vi "Demo2 (FPGA).vi"() -> ()   [LabVIEW 2023]
uses:
  Instance           1 20Saved   Demo2 (FPGA) .vi
  <vilib>/eio/EIONode/EIONode.xnode
  Instance           2 20Saved   Demo2 (FPGA) .vi
  <vilib>/rvi/DataTransferAndStorage/Container/XNode/niFpgaContainer.xnode
  <vilib>/rvi/eio/common/nirviEmuTemplateMethod_errors.vi
  <vilib>/rvi/FIFO/Fifo_Resource/nirvififoEmulationRead.vi
  <vilib>/rvi/FIFO/Fifo_Resource/nirvififoEmulationWrite.vi
panel:
  in  "Bypass interpolation filter?":bool
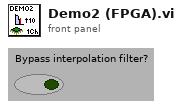
[diagram p1: front panel]
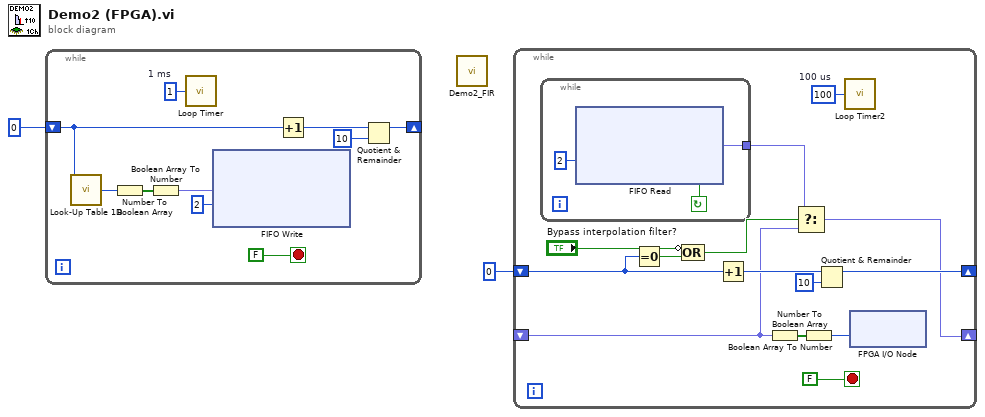
[diagram p0: block diagram]
diagram:
  n1 = while {
    shift-right: [w9] -> _
    shift-left: u8 0 -> [w8]
    stop <- FALSE stop-if-true
    w12 = u8 1  # 1 ms
    n2 = call "Look-Up Table 1D"("address"=w8) -> ("data out"=w7:i16)  [unwired: 8 in]
    n3 = Number To Boolean Array(number=w7) -> (Boolean array=w4:bool[])
    n4 = Boolean Array To Number(Boolean array=w4) -> (number=w3:fxp<+/-,16,1>)
    n5 = call "Loop Timer"("Count(mSec)"=w12) -> ()  [unwired: 1 out]
    n6 = xnode ("FIFO Write")("Element"=w3, "Timeout"=2) -> ()  [unwired: 1 in, 2 out]
    n7 = Increment(x=w8) -> (x+1=w11:u8)
    n8 = Quotient & Remainder(x=w11, y=u8 10) -> (x-y*floor(x/y)=w9:u8)  [unwired: 1 out]
  }
  n9 = call "Demo2_FIR.vi"() -> ()  [unwired: 1 out]
  n10 = while {
    shift-right: [w24] -> _
    shift-left: u8 0 -> [w23]
    shift-right: [w20] -> _
    shift-left: _ -> [w16]
    stop <- FALSE stop-if-true
    w17 = u8 100  # 100 us
    n11 = while {
      tunnel: [w28] -> w18
      stop <- w27 continue-if-true
      n12 = xnode ("FIFO Read")("Timeout"=2) -> ("Element"=w28:fxp<+/-,16,2>, "Timed Out?"=w27:bool)  [unwired: 1 in, 1 out]
    }
    n13 = Equal To 0?(x=w23) -> (x = 0?=w22:bool)
    n14 = Compound Arithmetic op=OR(invert "Bypass interpolation filter?", w22) -> (w15:bool)
    n15 = Increment(x=w23) -> (x+1=w26:u8)
    n16 = Number To Boolean Array(number=w16) -> (Boolean array=w14:bool[])
    n17 = Select(t=w18, s=w15, f=w16) -> (s? t:f=w20:fxp<+/-,16,2>)
    n18 = Boolean Array To Number(Boolean array=w14) -> (number=w13:i16)
    n19 = Quotient & Remainder(x=w26, y=u8 10) -> (x-y*floor(x/y)=w24:u8)  [unwired: 1 out]
    n20 = call "Loop Timer2"("Count(uSec)"=w17) -> ()  [unwired: 1 out]
    n21 = xnode "FPGA I/O Node"("AO0"=w13) -> ()  [unwired: 1 in, 1 out]
  }
